vi "Launch.vi"(8 "error in (no error)":errorcluster, 11 "comic_crawler in":refnum<class "comic_crawler.lvclass">) -> (0 "error out":errorcluster, 3 "comic_crawler out":refnum<class "comic_crawler.lvclass">)   [LabVIEW 2024, in "comic_crawler.lvclass"]
uses:
  comic_crawler.lvclass
  comic_crawler.lvclass/comic_crawler.ctl
  private/daemon.vi
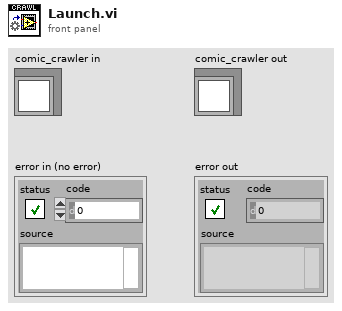
[diagram p1: front panel]
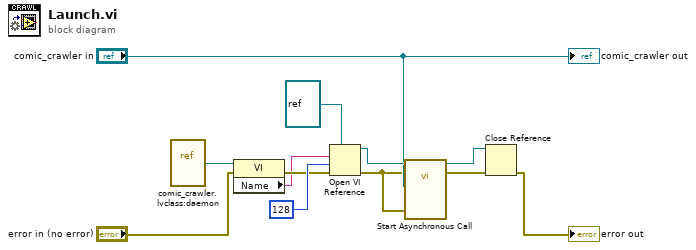
[diagram p0: block diagram]
diagram:
  n1 = vi-ref "comic_crawler.lvclass:daemon.vi"() -> (w11:refnum<vi>)
  n2 = property class="VI"(reference=w11, error in="error in (no error)") -> (error out=w10:errorcluster, "Name"=w9:string)  [unwired: 1 out]
  n3 = Open VI Reference(type specifier VI Refnum (for type only)=refnum<vi> refnum, vi path=w9, options=128, error in (no error)=w10) -> (vi reference=w7:refnum<vi>, error out=w1:errorcluster)  [unwired: 2 in]
  n4 = call-by-ref "Start Asynchronous Call"(reference=w7, error in=w1, 8:"error in (no error)"=w1, "comic_crawler.lvclass"="comic_crawler in") -> (reference out=w6:refnum<vi>, error out=w5:errorcluster)  [unwired: 10 in]
  n5 = Close Reference(reference=w6, error in (no error)=w5) -> (error out=→"error out":errorcluster)
  "comic_crawler out" <- "comic_crawler in"
